vi "create_analysis_plot.vi"(8 "error in (no error)":errorcluster, 10 "isotope name":string, 11 "Analysis in":refnum<class "Analysis.lvclass">) -> (0 "error out":errorcluster, 3 "PlotID out":string)   [LabVIEW 2015]
doc: "greates a plot for the selected isotope name ( item tag ) from the analysis data set. If Item tag is \"all\" a plot for each data set is created"
uses:
  MSControl/Classes/Analysis/Analysis.lvclass
  MSControl/Classes/Plots/Plots.lvclass
  global_variables.vi
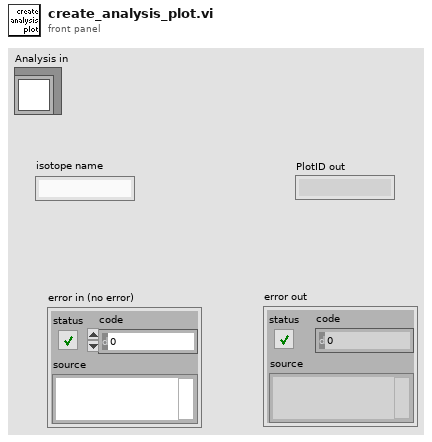
[diagram p1: front panel]
types:
  T1 = typedef "AnalysisDataArray.ctl" = cluster{"analysis data":string[][]}[]
  T2 = typedef "ExtrapolationResultsArray.ctl" = string[][]
  T3 = cluster{"format string":string, "Variant":variant}
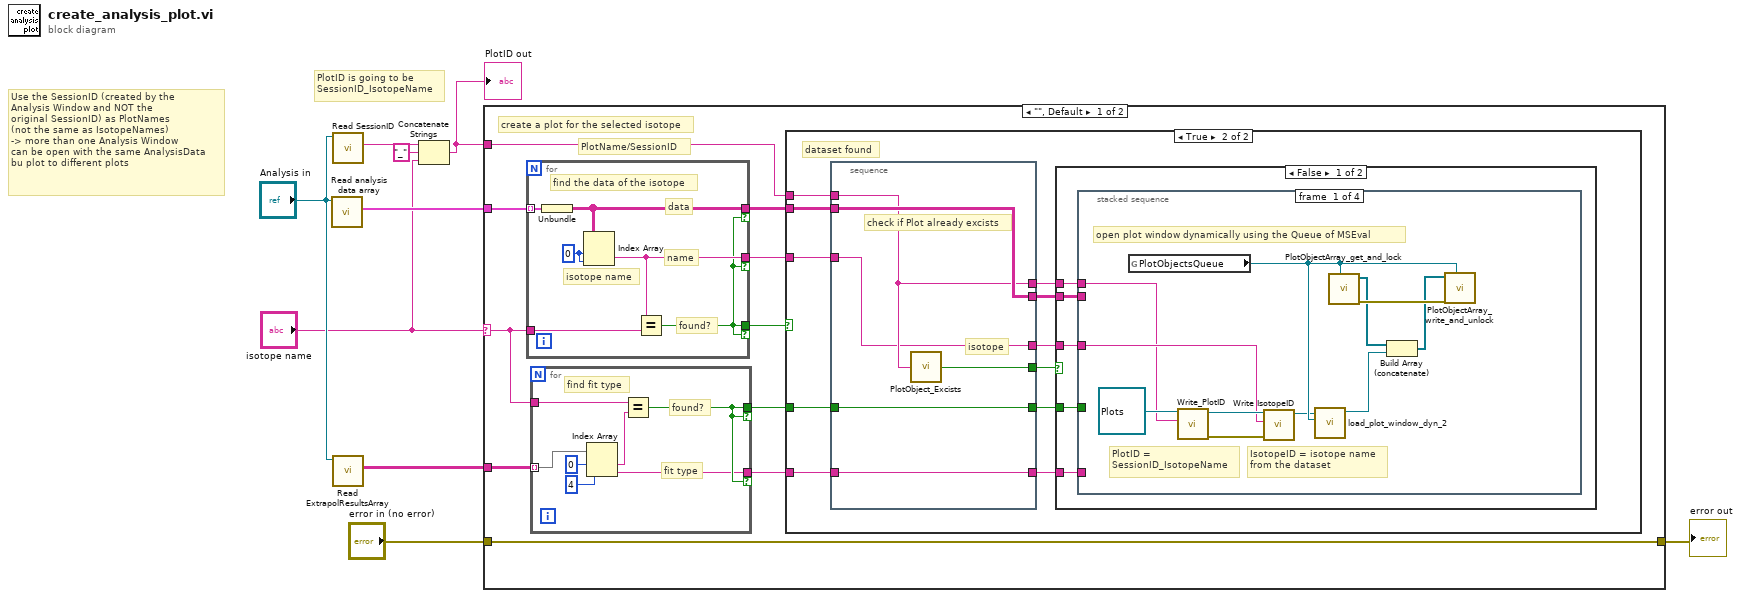
[diagram p0: block diagram]
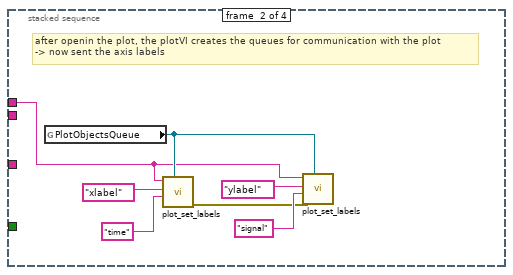
[diagram p3: hidden frame]
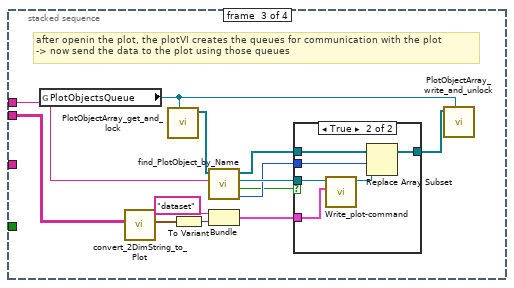
[diagram p4: hidden frame]
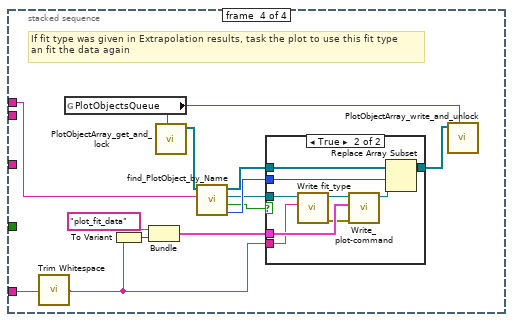
[diagram p6: hidden frame]
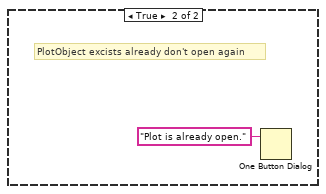
[diagram p8: hidden frame]
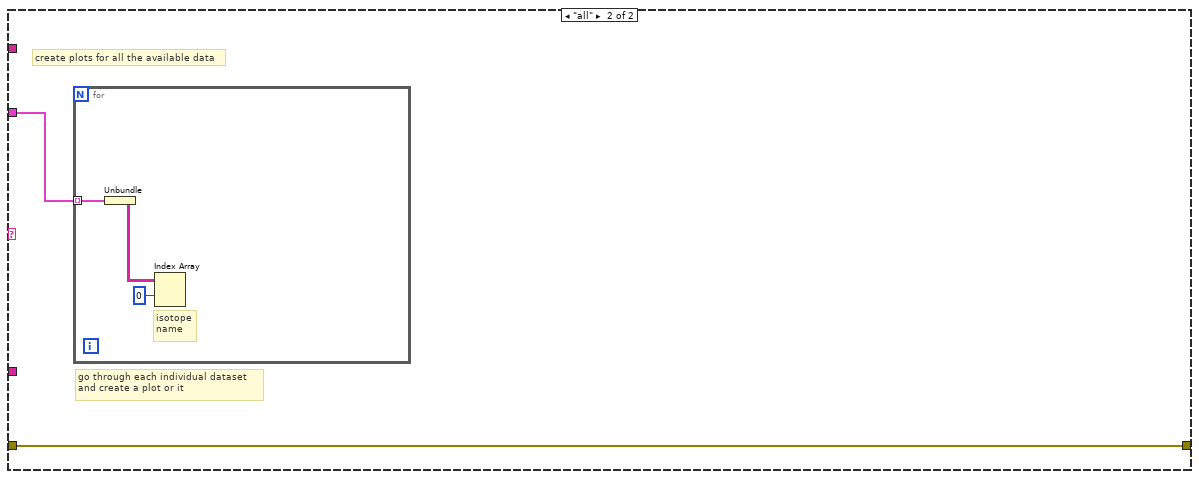
[diagram p9: hidden frame]
diagram:
  # "PlotID is going to be\nSessionID_IsotopeName"
  # "Use the SessionID (created by the\nAnalysis Window and NOT the\noriginal SessionID) as PlotNames\n(not the same as IsotopeNames)\n-> more than one Analysis Window\ncan be open with the same AnalysisData\nbu plot to different plots"
  n1 = call-dynamic "Read analysis data array.vi"("Analysis in"="Analysis in") -> ("analysis data array"=w9:T1)  [unwired: 8 in, 2 out]
  n2 = call-dynamic "Read SessionID.vi"("Analysis in"="Analysis in") -> ("SessionID"=w4:string)  [unwired: 8 in, 2 out]
  n3 = call-dynamic "Read ExtrapolResultsArray.vi"("Analysis in"="Analysis in") -> ("ExtrapolResultsArray"=w5:T2)  [unwired: 8 in, 2 out]
  n4 = Concatenate Strings(w4, "_" ("string"), "isotope name") -> (w3:string)
  "PlotID out" <- w3
  n5 = case shown="\"\", Default" "isotope name" {
    selector: "isotope name" -> [w12 _]
    tunnel: w9 -> [w19 w118]
    tunnel: "error in (no error)" -> [w15 w117]
    tunnel: [w15 w117] -> w7
    tunnel: w3 -> [w14 _]
    tunnel: w5 -> [w13 _]
    frame "", Default {
      # "PlotName/SessionID"
      # "create a plot for the selected isotope"
      n6 = for {
        tunnel: w12 -> [w114]
        tunnel: w19 -> [w116] mode=indexing
        tunnel: [w111] -> w18 if=w111
        tunnel: [w113] -> w17 if=w111
        tunnel: [w112] -> w16 if=w111
        w115 = 0 ("index (row)")
        # "find the data of the isotope"
        # "found?"
        # "name"
        # "data"
        # "isotope name"
        n7 = Unbundle(w116) -> ("analysis data"=w113:string[][])
        n8 = Index Array(array=w113, index (row)=w115, index (col)=w115) -> (element=w112:string)
        n9 = Equal?(x=w112, y=w114) -> (x = y?=w111:bool)
      }
      n10 = for {
        tunnel: w13 -> [w24] mode=indexing
        tunnel: w12 -> [w26]
        tunnel: [w20] -> w10 if=w23
        tunnel: [w23] -> w11 if=w23
        # "find fit type"
        # "found?"
        # "fit type"
        n11 = Index Array(array=w24, index #1=0 ("index"), index #2=4 ("index")) -> (element #1=w25:string, element #2=w20:string)
        n12 = Equal?(x=w26, y=w25) -> (x = y?=w23:bool)
      }
      n13 = case shown="True" w18 {
        tunnel: w17 -> [_ w35]
        tunnel: w16 -> [_ w33]
        tunnel: w14 -> [_ w37]
        tunnel: w11 -> [_ w30]
        tunnel: w10 -> [_ w29]
        frame False {
          # "no dataset found"
        }
        frame True {
          # "dataset found"
          n14 = stacked-sequence {
            tunnel: w37 -> [w108]
            tunnel: [w108] -> w36
            tunnel: w35 -> [w110]
            tunnel: [w110] -> w34
            tunnel: w33 -> [w105]
            tunnel: [w105] -> w32
            tunnel: [w109] -> w31
            tunnel: w30 -> [w107]
            tunnel: w29 -> [w106]
            tunnel: [w107] -> w28
            tunnel: [w106] -> w27
            frame #0 {
              # "isotope"
              # "check if Plot already excists"
              n15 = call "PlotObject_Excists.vi"("PlotName"=w108) -> ("found?"=w109:bool)
            }
          }
          n16 = case shown="False" w31 {
            tunnel: w36 -> [w42 _]
            tunnel: w34 -> [w41 _]
            tunnel: w32 -> [w40 _]
            tunnel: w28 -> [w39 _]
            tunnel: w27 -> [w38 _]
            frame False {
              n17 = stacked-sequence {
                tunnel: w40 -> [w44 _ _ _]
                tunnel: w41 -> [_ _ w66 _]
                tunnel: w42 -> [w43 w54 w62 w81]
                tunnel: w39 -> [_ _ _ _]
                tunnel: w38 -> [_ _ _ w84]
                frame #0 {
                  # "IsotopeID = isotope name\nfrom the dataset"
                  # "PlotID =\nSessionID_IsotopeName"
                  # "open plot window dynamically using the Queue of MSEval"
                  n18 = global read "global_variables.vi" "PlotObjectsQueue"() -> (w48:refnum<queue>)
                  n19 = call-dynamic "Write_PlotID.vi"("PlotID"=w43, "Plots in"=refnum<class "Plots.lvclass"> refnum ("Plots.lvclass")) -> ("error out"=w46:errorcluster, "Plots out"=w47:refnum<class "Plots.lvclass">)  [unwired: 8 in]
                  n20 = call-dynamic "Write IsotopeID.vi"("error in (no error)"=w46, "IsotopeID"=w44, "Plots in"=w47) -> ("Plots out"=w45:refnum<class "Plots.lvclass">)  [unwired: 7 in, 1 out]
                  n21 = call "load_plot_window_dyn_2.vi"("Ext PlotObjQueue in"=w48, "Plots in"=w45) -> ("Plots out"=w50:refnum<class "Plots.lvclass">)  [unwired: 8 in, 1 out]
                  n22 = call "PlotObjectArray_get_and_lock.vi"("External PlotObjQueue in"=w48) -> ("error out"=w53:errorcluster, "PlotObjects"=w51:refnum<class "Plots.lvclass">[])  [unwired: 9 in]
                  n23 = Build Array (concatenate)(w51, w50) -> (w49:refnum<class "Plots.lvclass">[])
                  n24 = call "PlotObjectArray_write_and_unlock.vi"("External PlotObjQueue in"=w48, "error in (no error)"=w53, "PlotObjects"=w49) -> ()  [unwired: 8 in, 1 out]
                }
                frame #1 {
                  # "after openin the plot, the plotVI creates the queues for communication with the plot\n-> now sent the axis labels"
                  n25 = global read "global_variables.vi" "PlotObjectsQueue"() -> (w55:refnum<queue>)
                  n26 = call "plot_set_labels.vi"("External PlotObjQueue in"=w55, "label"="time", "axis"="xlabel", "plot name"=w54) -> ("error out"=w56:errorcluster)  [unwired: 7 in]
                  n27 = call "plot_set_labels.vi"("External PlotObjQueue in"=w55, "error in (no error)"=w56, "label"="signal", "axis"="ylabel", "plot name"=w54) -> ()  [unwired: 6 in, 1 out]
                }
                frame #2 {
                  # "after openin the plot, the plotVI creates the queues for communication with the plot\n-> now send the data to the plot using those queues"
                  n28 = global read "global_variables.vi" "PlotObjectsQueue"() -> (w73:refnum<queue>)
                  n29 = call "convert_2DimString_to_Plot.vi"("string data in"=w66) -> ("Plot Data"=w64:cluster{dbl, dbl, "flag":u8}[])  [unwired: 9 in, 1 out]
                  n30 = call "PlotObjectArray_get_and_lock.vi"("External PlotObjQueue in"=w73) -> ("PlotObjects"=w72:refnum<class "Plots.lvclass">[])  [unwired: 9 in, 1 out]
                  n31 = To Variant(anything=w64) -> (Variant=w65:variant)
                  n32 = call "find_PlotObject_by_Name.vi"("Plot Name/ID"=w62, "PlotObj Array in"=w72) -> ("index of Object in Array"=w70:i32, "found?"=w61:bool, "found PlotObj out"=w71:refnum<class "Plots.lvclass">, "PlotObj Array out"=w69:refnum<class "Plots.lvclass">[])  [unwired: 6 in]
                  n33 = Bundle("format string"="dataset", "Variant"=w65) -> (w63:T3)  [unwired: 1 in]
                  n34 = case shown="True" w61 {
                    tunnel: w71 -> [_ w80]
                    tunnel: w70 -> [_ w78]
                    tunnel: w69 -> [w74 w77]
                    tunnel: [w74 w76] -> w68
                    tunnel: w63 -> [_ w75]
                    frame False {
                    }
                    frame True {
                      n35 = call-dynamic "Write_plot-command.vi"("plot command"=w75, "Plots in"=w80) -> ("Plots out"=w79:refnum<class "Plots.lvclass">)  [unwired: 8 in, 1 out]
                      n36 = Replace Array Subset(array=w77, new element=w79, index=w78) -> (w76:refnum<class "Plots.lvclass">[])
                    }
                  }
                  n37 = call "PlotObjectArray_write_and_unlock.vi"("External PlotObjQueue in"=w73, "PlotObjects"=w68) -> ()  [unwired: 9 in, 1 out]
                }
                frame #3 {
                  # "If fit type was given in Extrapolation results, task the plot to use this fit type\nan fit the data again"
                  n38 = call <vilib>:"Trim Whitespace.vi"("string"=w84) -> ("trimmed string"=w83:string)  [unwired: 1 in]
                  n39 = global read "global_variables.vi" "PlotObjectsQueue"() -> (w93:refnum<queue>)
                  n40 = To Variant(anything=w83) -> (Variant=w87:variant)
                  n41 = Bundle("format string"="plot_fit_data", "Variant"=w87) -> (w86:T3)  [unwired: 1 in]
                  n42 = call "PlotObjectArray_get_and_lock.vi"("External PlotObjQueue in"=w93) -> ("PlotObjects"=w92:refnum<class "Plots.lvclass">[])  [unwired: 9 in, 1 out]
                  n43 = call "find_PlotObject_by_Name.vi"("Plot Name/ID"=w81, "PlotObj Array in"=w92) -> ("index of Object in Array"=w91:i32, "found?"=w82:bool, "found PlotObj out"=w85:refnum<class "Plots.lvclass">, "PlotObj Array out"=w90:refnum<class "Plots.lvclass">[])  [unwired: 6 in]
                  n44 = case shown="True" w82 {
                    tunnel: w91 -> [_ w102]
                    tunnel: w90 -> [w94 w101]
                    tunnel: [w94 w100] -> w89
                    tunnel: w86 -> [_ w99]
                    tunnel: w85 -> [_ w98]
                    tunnel: w83 -> [_ w95]
                    frame False {
                    }
                    frame True {
                      n45 = call-dynamic "Write fit_type.vi"("fit_type"=w95, "Plots in"=w98) -> ("error out"=w96:errorcluster, "Plots out"=w97:refnum<class "Plots.lvclass">)  [unwired: 8 in]
                      n46 = call-dynamic "Write_plot-command.vi"("error in (no error)"=w96, "plot command"=w99, "Plots in"=w97) -> ("Plots out"=w103:refnum<class "Plots.lvclass">)  [unwired: 7 in, 1 out]
                      n47 = Replace Array Subset(array=w101, new element=w103, index=w102) -> (w100:refnum<class "Plots.lvclass">[])
                    }
                  }
                  n48 = call "PlotObjectArray_write_and_unlock.vi"("External PlotObjQueue in"=w93, "PlotObjects"=w89) -> ()  [unwired: 9 in, 1 out]
                }
              }
            }
            frame True {
              # "PlotObject excists already don't open again"
              n49 = One Button Dialog(message="Plot is already open.") -> ()  [unwired: 1 in, 1 out]
            }
          }
        }
      }
    }
    frame "all" {
      # "create plots for all the available data"
      # "go through each individual dataset\nand create a plot or it"
      n50 = for {
        tunnel: w118 -> [w121] mode=indexing
        # "isotope\nname"
        n51 = Unbundle(w121) -> ("analysis data"=w119:string[][])
        n52 = Index Array(array=w119, index (row)=0) -> ()  [unwired: 1 in, 1 out]
      }
    }
  }
  "error out" <- w7
